vi "Prosthetic Grasp.vi"   [LabVIEW 2016]
uses:
  <vilib>/NXT/Block Support/NXT_InputPort.ctl
  <vilib>/NXT/Block Support/NXT_ButtonSelector.ctl
  <vilib>/NXT/Block Support/NXT_OutputPort.ctl
  <vilib>/NXT/Dual Mode Library/Sensors/Touch_Count.vi
  <vilib>/NXT/Dual Mode Library/Display/drawNumber.vi
  <vilib>/NXT/NXTIO Xnodes/NXTIONodeSubVIs/NXTMoveMotors.vi
  <vilib>/NXT/Subs/LVHSConnector.ctl
  <vilib>/NXT/NXTIO Xnodes/AddressXNode/NXTIOAddress.xnode
  <vilib>/NXT/NXTIO Xnodes/NXTIOXNode/NXTIO.xnode
  <vilib>/NXT/Dual Mode Library/Sensors/readNXTButton.vi
  <vilib>/NXT/LegoClasses/BrickReference/BrickReference.lvclass
types:
  T1 = typedef "NXT_OutputPort.ctl" = u8
  T2 = typedef "NXT_ButtonSelector.ctl" = u16
  T3 = typedef "NXT_InputPort.ctl" = u32
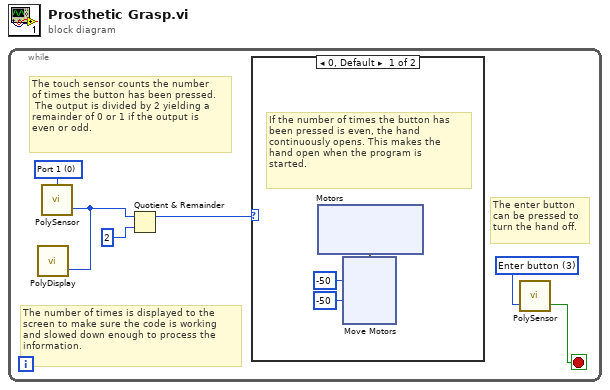
[diagram p0: block diagram]
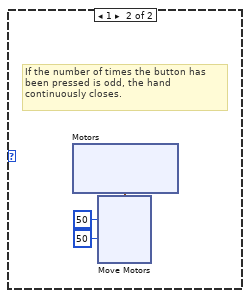
[diagram p2: hidden frame]
diagram:
  n1 = while {
    stop <- w3 stop-if-true
    w4 = T2 3 items=["Enter button"=3, "Left button"=2, "Right button"=1, "Up Button"=4, "Down Button"=5] ("Button (Enter button)")
    w6 = T3 0 items=["Port 1", "Port 2", "Port 3", "Port 4"] ("Port (Port 1)")
    # "The enter button\ncan be pressed to \nturn the hand off."
    # "The number of times is displayed to the \nscreen to make sure the code is working \nand slowed down enough to process the \ninformation."
    # "The touch sensor counts the number \nof times the button has been pressed.\n The output is divided by 2 yielding a \nremainder of 0 or 1 if the output is \neven or odd."
    n2 = call-poly <vilib>:"PolySensor.vi"("Port (Port 1)"=w6) -> ("Count"=w1:i16)  [unwired: 2 in, 1 out]
    n3 = call-poly <vilib>:"PolyDisplay.vi"("number"=w1) -> ()  [unwired: 3 in, 1 out]
    n4 = Quotient & Remainder(x=w1, y=i16 2) -> (x-y*floor(x/y)=w5:i16)  [unwired: 1 out]
    n5 = case shown="0, Default" w5 {
      frame 0, Default {
        # "If the number of times the button has \nbeen pressed is even, the hand \ncontinuously opens. This makes the \nhand open when the program is \nstarted."
        n6 = xnode "Motors"() -> ("Motor"=w9:cluster{"Port":T1, "Port":T1})
        n7 = xnode "Move Motors"("Power/Speed 2"=i8 -50, "Power/Speed 1"=i8 -50, "Motors"=w9) -> ()  [unwired: 1 in, 1 out]
      }
      frame 1 {
        # "If the number of times the button has \nbeen pressed is odd, the hand \ncontinuously closes."
        n8 = xnode "Motors"() -> ("Motor"=w21:cluster{"Port":T1, "Port":T1})
        n9 = xnode "Move Motors"("Power/Speed 2"=i8 50, "Power/Speed 1"=i8 50, "Motors"=w21) -> ()  [unwired: 1 in, 1 out]
      }
    }
    n10 = call-poly <vilib>:"PolySensor.vi"("Button (Enter button)"=w4) -> ("Yes/No"=w3:bool)  [unwired: 2 in, 1 out]
  }
